vi "Initialise Observers.vi"(8 "error in (no error)":errorcluster, 11 "Main Controller in":refnum<class "Main Controller Actor.lvclass">) -> (0 "error out":errorcluster, 3 "Main Controller out":refnum<class "Main Controller Actor.lvclass">, 5 "Observers":cluster{"Actor":refnum<event-registration>})   [LabVIEW 2021, in "Main Controller Actor.lvclass"]
uses:
  Main Controller Actor.lvclass
  Main Controller Actor.lvclass/Main Controller Actor.ctl
  Re-use Libraries/Minimal Actor Framework/Messaging/Message/Message.lvclass
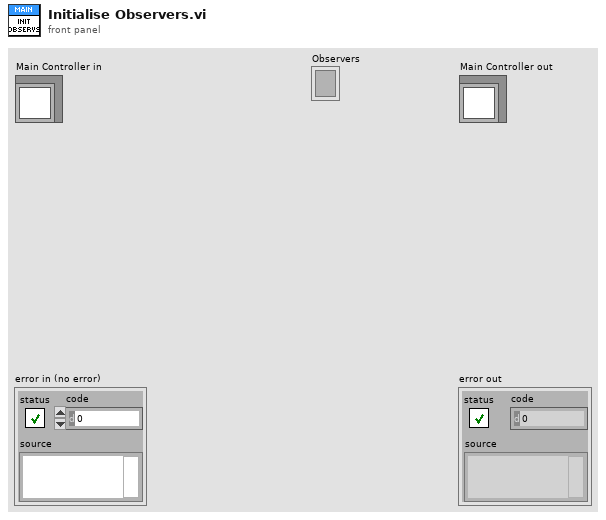
[diagram p1: front panel]
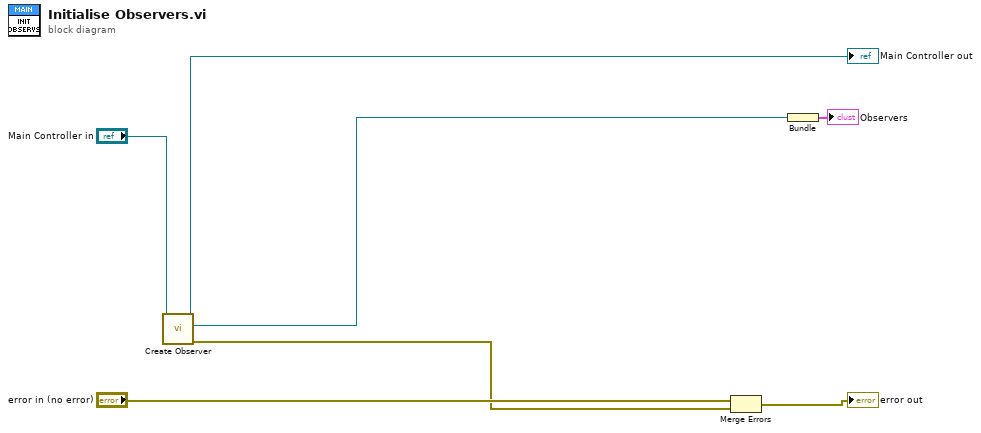
[diagram p0: block diagram]
diagram:
  n1 = call-dynamic "Create Observer.vi"("Actor in"="Main Controller in") -> ("error out"=w3:errorcluster, "Actor"=w6:refnum<event-registration>, "Actor out"=→"Main Controller out":refnum<class "Main Controller Actor.lvclass">)  [unwired: 8 in]
  n2 = Merge Errors("error in (no error)", w3) -> (→"error out":errorcluster)
  n3 = Bundle("Actor"=w6) -> (→"Observers":cluster{"Actor":refnum<event-registration>})  [unwired: 1 in]
